vi "AFM_sync_fixed_lightsheet_new.vi"() -> ()   [LabVIEW 2017]
uses:
  <vilib>/DAQmx/write.llb/DAQmx Write (Analog DBL 1Chan 1Samp).vi
  <vilib>/DAQmx/write.llb/DAQmx Write (Analog 2D DBL NChan NSamp).vi
  <vilib>/DAQmx/create/channels.llb/DAQmx Create Channel (AO-Voltage-Basic).vi
  <vilib>/DAQmx/miscellaneous.llb/DAQmx Fill In Error Info.vi
  <vilib>/DAQmx/configure/timing.llb/DAQmx Timing (Sample Clock).vi
  <vilib>/DAQmx/configure/trigger.llb/DAQmx Start Trigger (Digital Edge).vi
  <resource>/objmgr/daqmx.rc
panel:
  out "Matched AFM Frequency (Hz)":dbl
  in  "ETL3 (V)  (4.76V allows light passing through unaltered.)":dbl(slide)=4.76 caption="ETL3 (dpt)" min=-12.029999732971191 max=16.450000762939453 step=0.009999999776482582 scale=0.0..10.0
  out "Focal Distance (um)":dbl
  out "Diopter":dbl
  in  "561 Intensity (0-10v)":dbl=3.0
  in  "488 Intensity (0-10v)":dbl=3.0
  in  "Off Time (ms)":dbl=100.0
  in  "On Time (ms)":dbl=300.0
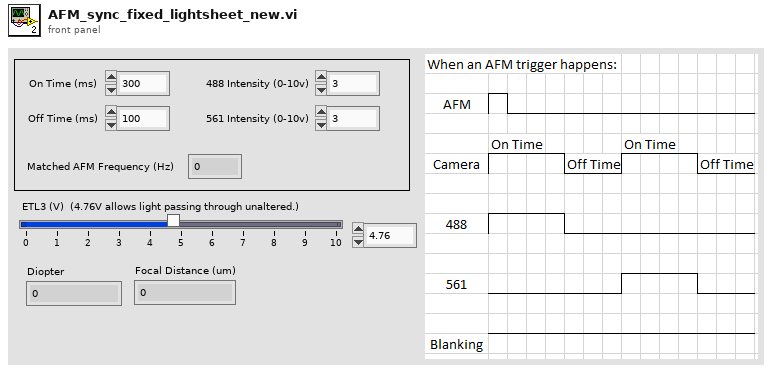
[diagram p1: front panel]
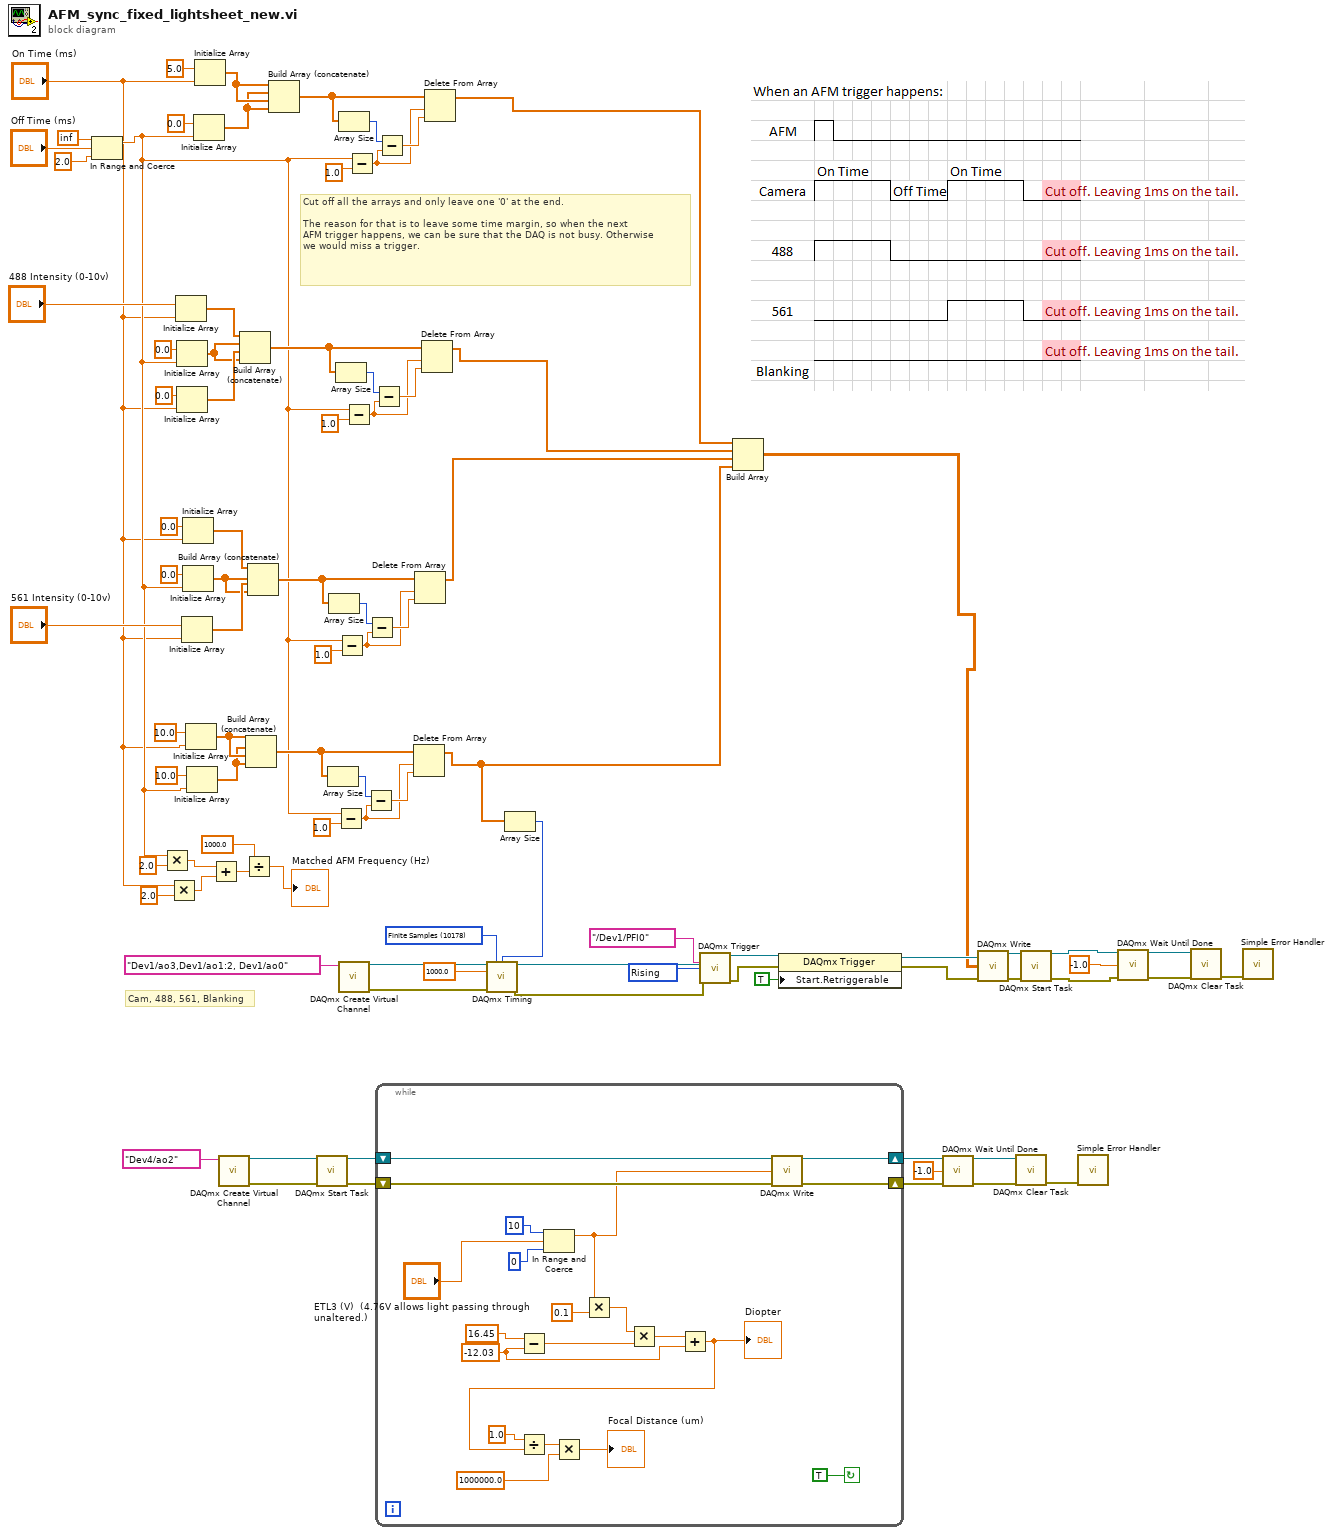
[diagram p0: block diagram]
diagram:
  w25 = 10280 items=["Rising"=10280, "Falling"=10171] ("edge")
  w37 = 10178 items=["Finite Samples"=10178, "Continuous Samples"=10123, "Hardware Timed Single Point"=12522] ("sample mode")
  # "Cut off all the arrays and only leave one '0' at the end.\n\nThe reason for that is to leave some time margin, so when the next \nAFM trigger happens, we can be sure that the DAQ is not busy. Otherwise\nwe would miss a trigger."
  # "Cam, 488, 561, Blanking"
  n1 = In Range and Coerce(upper limit=inf, x="Off Time (ms)", lower limit=2.0) -> (coerced(x)=w16:dbl)  [unwired: 1 out]
  n2 = Multiply(x=w16, y=2.0) -> (x*y=w11:dbl)
  n3 = Multiply(x="On Time (ms)", y=2.0) -> (x*y=w12:dbl)
  n4 = Initialize Array("488 Intensity (0-10v)", "On Time (ms)") -> (w65:dbl[])
  n5 = Initialize Array(0.0 ("element"), w16) -> (w63:dbl[])
  n6 = Initialize Array(0.0 ("element"), "On Time (ms)") -> (w64:dbl[])
  n7 = Initialize Array("561 Intensity (0-10v)", "On Time (ms)") -> (w53:dbl[])
  n8 = Initialize Array(0.0 ("element"), "On Time (ms)") -> (w54:dbl[])
  n9 = Initialize Array(0.0 ("element"), w16) -> (w52:dbl[])
  n10 = Initialize Array(10.0 ("element"), "On Time (ms)") -> (w44:dbl[])
  n11 = Initialize Array(10.0 ("element"), w16) -> (w17:dbl[])
  n12 = Initialize Array(0.0 ("element"), w16) -> (w74:dbl[])
  n13 = Initialize Array(5.0 ("element"), "On Time (ms)") -> (w75:dbl[])
  n14 = Add(x=w11, y=w12) -> (x+y=w10:dbl)
  n15 = call-poly <vilib>:"DAQmx Create Virtual Channel.vi"("physical channels"=tag "Dev4/ao2") -> ("task out"=w84:refnum<k21>, "error out"=w83:errorcluster)  [unwired: 13 in]
  n16 = Build Array (concatenate)(w65, w63, w64, w63) -> (w58:dbl[])
  n17 = Divide(x=1000.0, y=w10) -> (x/y=→"Matched AFM Frequency (Hz)":dbl)
  n18 = Build Array (concatenate)(w44, w17, w44, w17) -> (w39:dbl[])
  n19 = Build Array (concatenate)(w54, w52, w53, w52) -> (w47:dbl[])
  n20 = Build Array (concatenate)(w75, w74, w75, w74) -> (w73:dbl[])
  n21 = call <vilib>:"DAQmx Start Task.vi"("task/channels in"=w84, "error in"=w83) -> ("task out"=w86:refnum<k21>, "error out"=w85:errorcluster)  [unwired: 12 in]
  n22 = Array Size(array=w39) -> (size(s)=w43:i32)
  n23 = Array Size(array=w47) -> (size(s)=w51:i32)
  n24 = Array Size(array=w58) -> (size(s)=w62:i32)
  n25 = Subtract(x=w16, y=1.0) -> (x-y=w40:dbl)
  n26 = Subtract(x=w16, y=1.0) -> (x-y=w48:dbl)
  n27 = Array Size(array=w73) -> (size(s)=w72:i32)
  n28 = call-poly <vilib>:"DAQmx Create Virtual Channel.vi"("physical channels"=tag "Dev1/ao3,Dev1/ao1:2, Dev1/ao0") -> ("task out"=w28:refnum<k21>, "error out"=w27:errorcluster)  [unwired: 13 in]
  n29 = Subtract(x=w16, y=1.0) -> (x-y=w59:dbl)
  n30 = Subtract(x=w16, y=1.0) -> (x-y=w69:dbl)
  n31 = Subtract(x=w43, y=w40) -> (x-y=w41:dbl)
  n32 = Subtract(x=w51, y=w48) -> (x-y=w49:dbl)
  n33 = Subtract(x=w62, y=w59) -> (x-y=w60:dbl)
  n34 = while {
    shift-right: [w109] -> w81
    shift-left: w86 -> [w111]
    shift-right: [w108] -> w82
    shift-left: w85 -> [w110]
    stop <- TRUE continue-if-true
    w93 = -12.03 ("x")
    n35 = Subtract(x=16.45 ("y"), y=w93) -> (x-y=w95:dbl)
    n36 = In Range and Coerce(upper limit=10, x="ETL3 (V)  (4.76V allows light passing through unaltered.)", lower limit=0) -> (coerced(x)=w98:dbl)  [unwired: 1 out]
    n37 = Multiply(x=w98, y=0.1) -> (x*y=w96:dbl)
    n38 = Multiply(x=w96, y=w95) -> (x*y=w94:dbl)
    n39 = Add(x=w94, y=w93) -> (x+y=w92:dbl)
    "Diopter" <- w92
    n40 = Divide(x=1.0, y=w92) -> (x/y=w105:dbl)
    n41 = Multiply(x=w105, y=1000000.0) -> (x*y=→"Focal Distance (um)":dbl)
    n42 = call-poly <vilib>:"DAQmx Write.vi"("task/channels in"=w111, "data"=w98, "error in"=w110) -> ("task out"=w109:refnum<k21>, "error out"=w108:errorcluster)  [unwired: 10 in, 1 out]
  }
  n43 = Subtract(x=w72, y=w69) -> (x-y=w70:dbl)
  n44 = Delete From Array(array=w39, length=w40, index=w41) -> (array with subset deleted=w2:dbl[])  [unwired: 1 out]
  n45 = Delete From Array(array=w47, length=w48, index=w49) -> (array with subset deleted=w5:dbl[])  [unwired: 1 out]
  n46 = Delete From Array(array=w58, length=w59, index=w60) -> (array with subset deleted=w6:dbl[])  [unwired: 1 out]
  n47 = Delete From Array(array=w73, length=w69, index=w70) -> (array with subset deleted=w7:dbl[])  [unwired: 1 out]
  n48 = Array Size(array=w2) -> (size(s)=w1:i32)
  n49 = call-poly <vilib>:"DAQmx Timing.vi"("task/channels in"=w28, "sample mode"=w37, "samples per channel"=w1, "rate"=1000.0, "error in"=w27) -> ("task out"=w24:refnum<k21>, "error out"=w23:errorcluster)  [unwired: 9 in]
  n50 = call-poly <vilib>:"DAQmx Trigger.vi"("task/channels in"=w24, "source"=tag "/Dev1/PFI0", "edge"=w25, "error in"=w23) -> ("task out"=w21:refnum<k21>, "error out"=w18:errorcluster)  [unwired: 10 in]
  n51 = Build Array(w7, w6, w5, w2) -> (w3:dbl[][])
  n52 = property class="DAQmx Trigger"(reference=w21, error in=w18, "Start.Retriggerable"=TRUE) -> (reference out=w20:refnum<k21>, error out=w19:errorcluster)
  n53 = call <vilib>:"DAQmx Wait Until Done.vi"("task/channels in"=w81, "timeout (sec)"=-1.0, "error in"=w82) -> ("task out"=w90:refnum<k21>, "error out"=w89:errorcluster)  [unwired: 11 in]
  n54 = call-poly <vilib>:"DAQmx Write.vi"("task/channels in"=w20, "data"=w3, "error in"=w19) -> ("task out"=w31:refnum<k21>, "error out"=w30:errorcluster)  [unwired: 10 in, 1 out]
  n55 = call <vilib>:"DAQmx Clear Task.vi"("task in"=w90, "error in"=w89) -> ("error out"=w91:errorcluster)  [unwired: 13 in]
  n56 = call <vilib>:"DAQmx Start Task.vi"("task/channels in"=w31, "error in"=w30) -> ("task out"=w33:refnum<k21>, "error out"=w34:errorcluster)  [unwired: 12 in]
  n57 = call <vilib>:"Simple Error Handler.vi"("error in (no error)"=w91) -> ()  [unwired: 4 in, 5 out]
  n58 = call <vilib>:"DAQmx Wait Until Done.vi"("task/channels in"=w33, "timeout (sec)"=-1.0, "error in"=w34) -> ("task out"=w36:refnum<k21>, "error out"=w35:errorcluster)  [unwired: 11 in]
  n59 = call <vilib>:"DAQmx Clear Task.vi"("task in"=w36, "error in"=w35) -> ("error out"=w38:errorcluster)  [unwired: 13 in]
  n60 = call <vilib>:"Simple Error Handler.vi"("error in (no error)"=w38) -> ()  [unwired: 4 in, 5 out]
